vi "Saving Time.vi"(6 "File Save Time":string, 8 "error in (no error)":errorcluster) -> (0 "error out":errorcluster)   [LabVIEW 2021]
uses:
  <vilib>/Utility/file.llb/Write Delimited Spreadsheet (string).vi
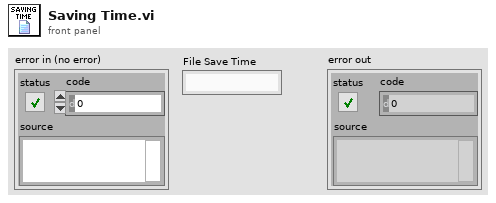
[diagram p1: front panel]
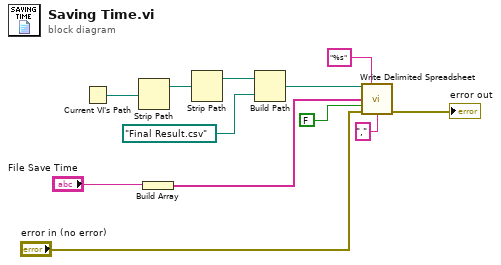
[diagram p0: block diagram]
diagram:
  n1 = Current VI's Path() -> (path=w11:path)
  n2 = Strip Path(path=w11) -> (stripped path=w12:path)  [unwired: 1 out]
  n3 = Build Array("File Save Time") -> (w3:string[])
  n4 = Strip Path(path=w12) -> (stripped path=w10:path)  [unwired: 1 out]
  n5 = Build Path(base path=w10, name or relative path=path "Final Result.csv") -> (appended path=w8:path)
  n6 = call-poly <vilib>:"Write Delimited Spreadsheet.vi"("file path (dialog if empty)"=w8, "format (%s)"="%s", "1D data"=w3, "append to file? (new file:F)"=FALSE, "error in (no error)"="error in (no error)", "delimiter (\\t)"="," ("delimiter (\\t)")) -> ("error out"=→"error out":errorcluster)  [unwired: 8 in, 1 out]
